vi "Read Data Map.vi"(8 "error in":errorcluster, 11 "Controller in":refnum<class "Controller.lvclass">) -> (0 "error out":errorcluster, 2 "MAP DVR":refnum<data-value>, 3 "Controller out":refnum<class "Controller.lvclass">)   [LabVIEW 2014, in "Controller.lvlib" / "Controller.lvclass"]
uses:
  Controller.lvclass
  Controller.lvclass/Controller.ctl
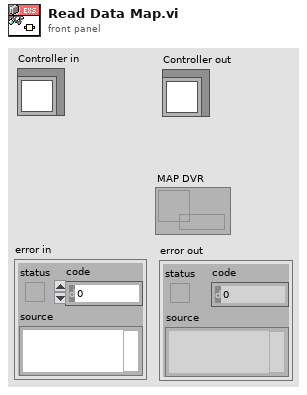
[diagram p1: front panel]
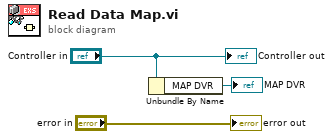
[diagram p0: block diagram]
diagram:
  n1 = Unbundle By Name("Controller in") -> ("MAP DVR"=→"MAP DVR":refnum<data-value>)
  "error out" <- "error in"
  "Controller out" <- "Controller in"
